vi "GetScanTime.vi"(8 "error in (no error)":errorcluster caption="entrée d'erreur (pas d'erreur)", 11 "Experiment en entrée":refnum<class "Experiment.lvclass"> caption="DNL_LabVIEW Object in") -> (0 "error out":errorcluster caption="sortie d'erreur", 2 "NbPos":i32, 3 "Experiment en sortie":refnum<class "Experiment.lvclass"> caption="DNL_LabVIEW Object out")   [LabVIEW 2019, in "Experiment.lvclass"]
uses:
  Experiment.lvclass
  Experiment.lvclass/Experiment.ctl
  DevicesClass/BaseDevice/BaseDevice.lvclass
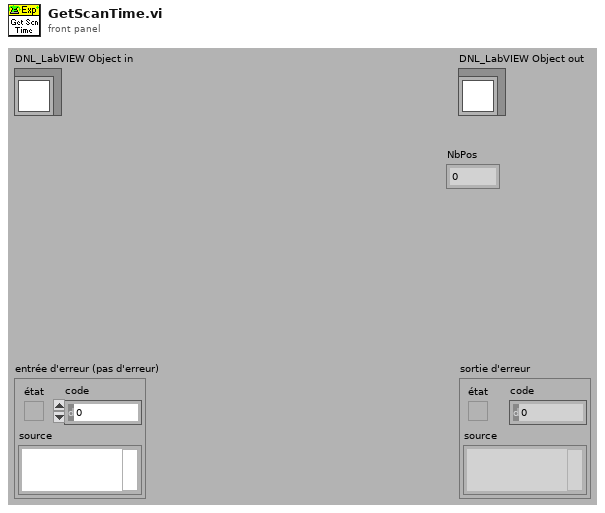
[diagram p1: front panel]
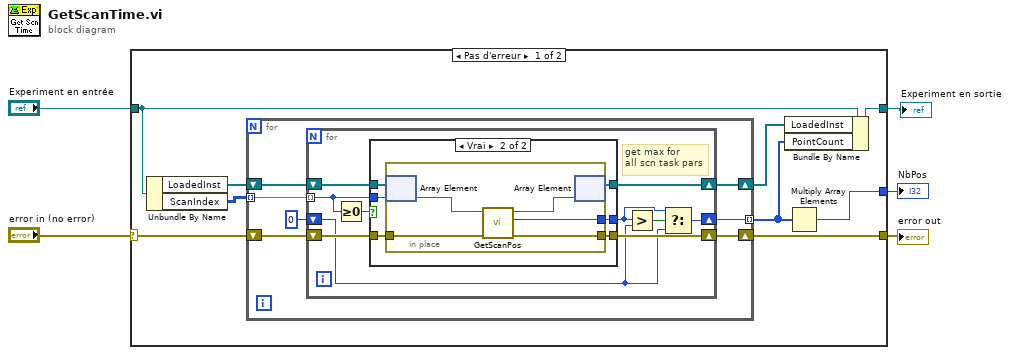
[diagram p0: block diagram]
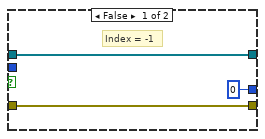
[diagram p2: hidden frame]
diagram:
  n1 = case shown="Pas d'erreur" "error in (no error)" {
    selector: "error in (no error)" -> [w11 w47]
    tunnel: [w8 w47] -> w4
    tunnel: [w12 w46] -> w2
    tunnel: "Experiment en entrée" -> [w14 w46]
    tunnel: [w6 _] -> w1
    frame No Error {
      n2 = Unbundle By Name(w14) -> ("LoadedInst"=w13:refnum<class "BaseDevice.lvclass">[], "ScanIndex"=w10:i32[][])
      n3 = for {
        tunnel: [w16] -> w7 mode=indexing
        tunnel: w10 -> [w19] mode=indexing
        shift-right: [w18] -> w9
        shift-left: w13 -> [w21]
        shift-right: [w17] -> w8
        shift-left: w11 -> [w20]
        n4 = for {
          tunnel: w19 -> [w23] mode=indexing
          shift-right: [w30] -> w18
          shift-left: w21 -> [w31]
          shift-right: [w28] -> w17
          shift-left: w20 -> [w29]
          shift-right: [w25] -> w16
          shift-left: 0 ("nb pos") -> [w22]
          # "get max for \nall scn task pars"
          n5 = Greater Or Equal To 0?(x=w23) -> (x >= 0?=w24:bool)
          n6 = case shown="Vrai" w24 {
            tunnel: w31 -> [w34 w40]
            tunnel: w23 -> [_ w39]
            tunnel: [w34 w38] -> w30
            tunnel: w29 -> [w33 w37]
            tunnel: [w33 w36] -> w28
            tunnel: [0 ("nb pos") w35] -> w26
            frame False {
              # "Index = -1"
            }
            frame True {
              n7 = in-place {
                in-place-border: w37 -> [w44]
                in-place-border: [w41] -> w35
                in-place-border: [w43] -> w36
                n8 = in-place-array #1(w40, w39) -> (w45:refnum<class "BaseDevice.lvclass">)
                n9 = call "GetScanPos.vi"("error in (no error)"=w44, "BaseDevice en entrée"=w45) -> ("error out"=w43:errorcluster, "nb pos"=w41:i32, "BaseDevice en sortie"=w42:refnum<class "BaseDevice.lvclass">)  [unwired: 4 in, 3 out]
                n10 = in-place-array #1(w42) -> (w38:refnum<class "BaseDevice.lvclass">[])  [unwired: 1 out]
              }
            }
          }
          n11 = Greater?(x=w26, y=w22) -> (0:w27:bool)
          n12 = Select(t=w26, s=w27, f=w22) -> (s? t:f=w25:i32)
        }
      }
      n13 = Bundle By Name(cluster=w14, "LoadedInst"=w9, "PointCount"=w7) -> (w12:refnum<class "Experiment.lvclass">)
      n14 = Multiply Array Elements(1:w7) -> (0:w6:i32)
    }
    frame Error {
    }
  }
  "error out" <- w4
  "Experiment en sortie" <- w2
  "NbPos" <- w1
